vi "Find Root of f_W,T,D(x) = 0.vi"(4 "data":variant, 5 "x":dbl) -> (2 "f(x)":dbl)   [LabVIEW 2019]
uses:
  Square Gated 1-Exp Parameters.ctl
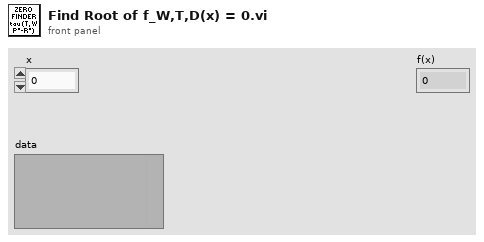
[diagram p1: front panel]
types:
  T1 = typedef "Square Gated 1-Exp Parameters.ctl" = cluster{"P-R":dbl, "W":dbl, "T":dbl}
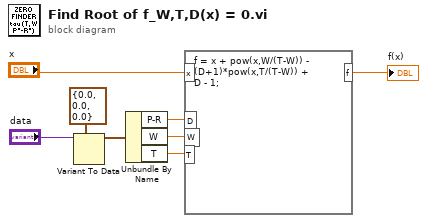
[diagram p0: block diagram]
diagram:
  n1 = Variant To Data(type=T1 {"P-R"=0.0, "W"=0.0, "T"=0.0} ("output cluster"), Variant="data") -> (data=w6:T1)  [unwired: 1 in, 1 out]
  n2 = Unbundle By Name(w6) -> ("P-R"=w5:dbl, "W"=w4:dbl, "T"=w3:dbl)
  n3 = formula code="f = x + pow(x,W/(T-W)) -\n(D+1)*pow(x,T/(T-W)) +\nD - 1;"("D"=w5, "W"=w4, "T"=w3, "x"="x") -> ("f"=→"f(x)":dbl)
